vi "单通道循环读取.vi"(7 "超时s":dbl=1.5, 8 "error in (no error)":errorcluster caption="错误输入（无错误）", 9 "分析仪通道":T1(ring), 10 "地址":string="02", 11 "MyIndex":u8) -> (0 "error out":errorcluster caption="错误输出", 2 "通道数据":u16[](array[numeric]), 3 "循环数据":u16[][](array[numeric]))   [LabVIEW 2015]
uses:
  <vilib>/Instr/_visa.llb/VISA Configure Serial Port (Instr).vi
panel:
  out "Read":string
  out "Send":string
  # "R"
  # "G"
  # "B"
  # "i"
  # "H"
  # "S"
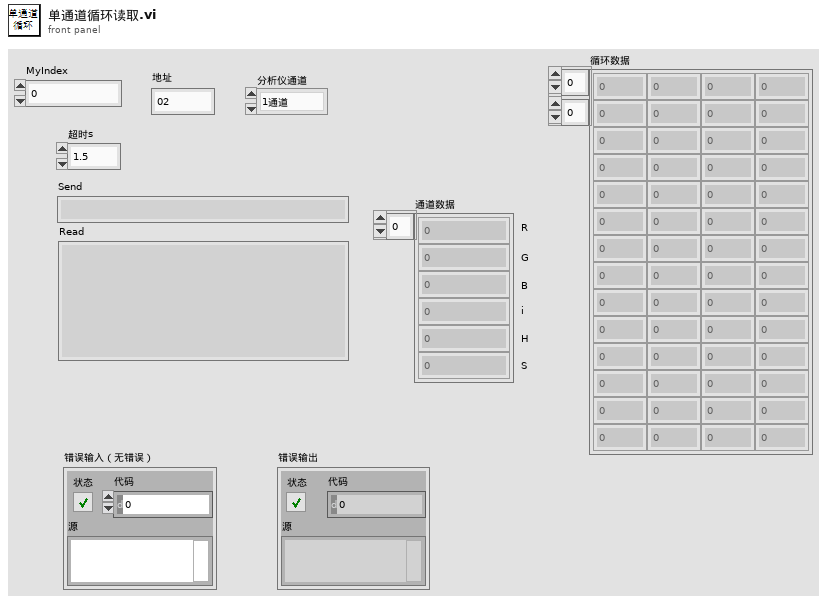
[diagram p1: front panel]
types:
  T1 = enum16{"1通道", "2通道", "3通道", "4通道", "5通道", "6通道", "7通道", "8通道", "9通道", "10通道", "11通道", "12通道", "13通道", "14通道", "15通道", "16通道"}
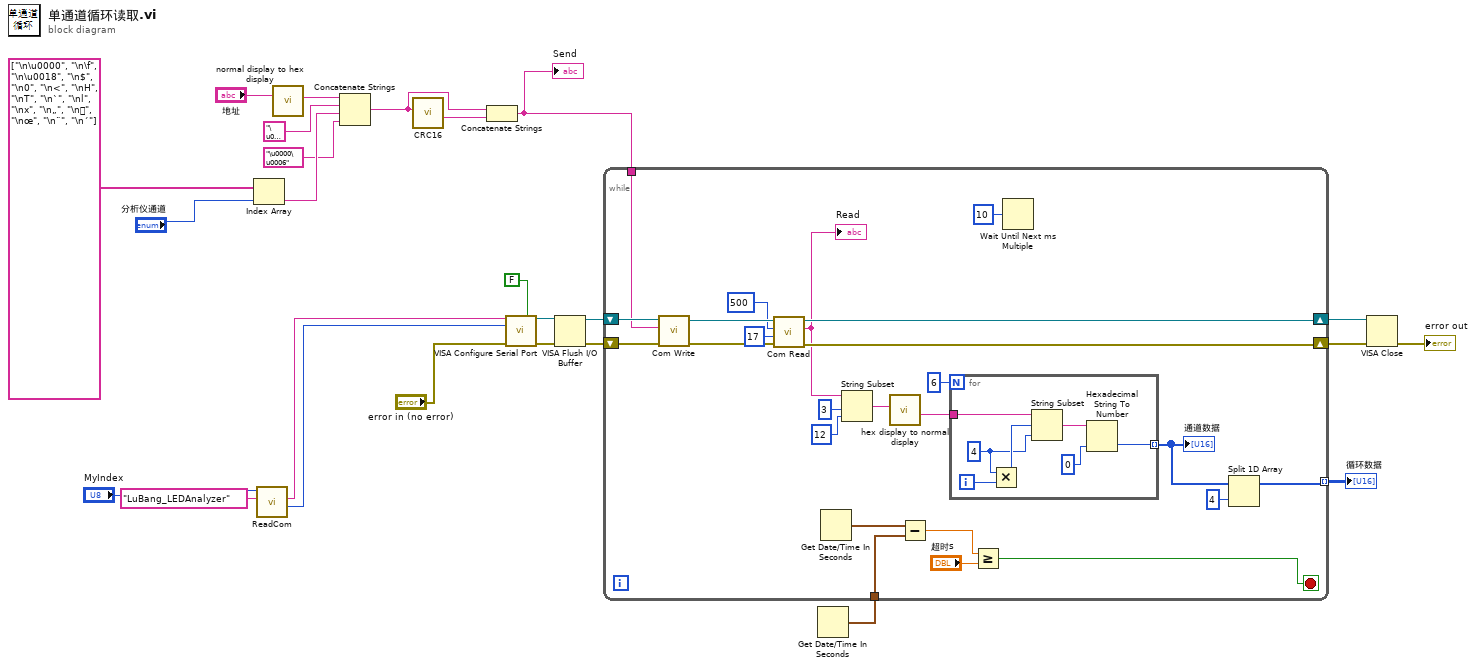
[diagram p0: block diagram]
diagram:
  n1 = Index Array(array=string[] ["\n\u0000", "\n\f", "\n\u0018", "\n$", "\n0", "\n<", "\nH", "\nT", "\n`", "\nl", "\nx", "\n„", "\n", "\nœ", "\n¨", "\n´"], index="分析仪通道") -> (element=w14:string)
  n2 = call "ReadCom.vi"("仪器名称"="LuBang_LEDAnalyzer", "MyIndex"="MyIndex") -> ("Baudrate"=w1:i32, "COM"=w2:string)  [unwired: 7 in, 1 out]
  n3 = call "normal display to hex display.vi"("Normal display"="地址") -> ("Hex display"=w18:string)  [unwired: 6 in]
  n4 = Concatenate Strings(w18, "\u0003", w14, "\u0000\u0006") -> (w22:string)
  n5 = call "CRC16.vi"("输入字符串"=w22) -> ("CRC16(String)"=w21:string)  [unwired: 9 in, 1 out]
  n6 = Concatenate Strings(w22, w21) -> (w10:string)
  "Send" <- w10
  n7 = call-poly "VISA Configure Serial Port"("VISA resource name"=w2, "Enable Termination\nChar (T)"=FALSE ("Enable Termination\nChar (T)"), "baud rate (9600)"=w1, "error in (no error)"="error in (no error)") -> ("VISA resource name out"=w23:refnum<visa-resource-name>, "error out"=w24:errorcluster)  [unwired: 10 in]
  n8 = VISA Flush I/O Buffer(VISA resource name=w23, error in (no error)=w24) -> (VISA resource name out=w12:refnum<visa-resource-name>, error out=w11:errorcluster)  [unwired: 1 in]
  n9 = Get Date/Time In Seconds() -> (seconds since 1Jan1904=w5:timestamp)
  n10 = while {
    tunnel: w10 -> [w47]
    shift-right: [w42] -> w9
    shift-left: w12 -> [w49]
    shift-right: [w41] -> w8
    shift-left: w11 -> [w48]
    tunnel: [w32] -> w6 mode=indexing
    tunnel: w5 -> [w30]
    stop <- w27 stop-if-true
    n11 = call "Com Write.vi"("错误输入（无错误）"=w48, "Wbuff"=w47, "VISA In"=w49) -> ("错误输出"=w46:errorcluster, "VISA Out"=w45:refnum<visa-resource-name>)  [unwired: 7 in]
    n12 = call "Com Read.vi"("错误输入（无错误）"=w46, "num"=u32 17, "超时"=u32 500, "VISA In"=w45) -> ("错误输出"=w41:errorcluster, "buff"=w40:string, "VISA Out"=w42:refnum<visa-resource-name>)  [unwired: 5 in]
    "Read" <- w40
    n13 = Get Date/Time In Seconds() -> (seconds since 1Jan1904=w31:timestamp)
    n14 = String Subset(string=w40, offset (0)=3 ("长度（剩余）"), length (rest)=12 ("长度（剩余）")) -> (substring=w37:string)
    n15 = call "hex display to normal display.vi"("Hex display"=w37) -> ("Normal display"=w36:string)  [unwired: 10 in]
    n16 = Subtract(x=w31, y=w30) -> (x-y=w29:dbl)
    n17 = for {
      N: 6 -> [_]
      tunnel: w36 -> [w56]
      tunnel: [w51] -> w33 mode=indexing
      i -> [w55]
      w53 = 4
      n18 = Multiply(x=w53, y=w55) -> (x*y=w54:i32)
      n19 = String Subset(string=w56, offset (0)=w54, length (rest)=w53) -> (substring=w52:string)
      n20 = Hexadecimal String To Number(string=w52, default (0uL)=u16 0) -> (number=w51:u16)  [unwired: 1 in, 1 out]
    }
    "通道数据" <- w33
    n21 = Greater Or Equal?(x=w29, y="超时s") -> (x >= y?=w27:bool)
    n22 = Wait Until Next ms Multiple(millisecond multiple=u32 10 ("毫秒倍数")) -> ()  [unwired: 1 out]
    n23 = Split 1D Array(array=w33, index=4 ("索引")) -> (first subarray=w32:u16[])  [unwired: 1 out]
  }
  "循环数据" <- w6
  n24 = VISA Close(VISA resource name=w9, error in (no error)=w8) -> (error out=→"error out":errorcluster)
